vi "LINX - Servo Puerta 2.vi"() -> ()   [LabVIEW 2019]
doc: "This example demonstrates how to control a servo using LINX."
uses:
  <vilib>/MakerHub/LINX/Public/Utilities/Open Serial.vi
  <vilib>/MakerHub/LINX/Public/Sensors/Motion/Servo/Servo Open One Channel.vi
  <vilib>/MakerHub/LINX/Public/Sensors/Motion/Servo/Servo Set Pulse Width One Channel.vi
  <vilib>/MakerHub/LINX/Public/Sensors/Motion/Servo/Servo Close One Channel.vi
  <vilib>/MakerHub/LINX/LMH-LINX.lvlib
  <vilib>/MakerHub/LINX/Public/Sensors/Motion/Servo/Servo.lvlib
panel:
  out "Loop Rate (Hz)":u32
  in  "Cerrar":bool
  in  "Abrir":bool
  in  "Servo Channel":u8=2
  in  "Stop Button":bool
  in  "Serial Port":refnum<visa-resource-name>
  # "Servo Position \n(Pulse Width uS)"
  # "LINX Device Settings"
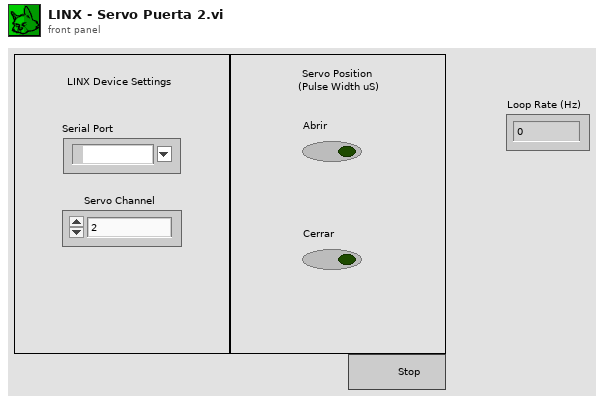
[diagram p1: front panel]
types:
  T1 = typedef "LMH-LINX.lvlib/LINX Ref.ctl" = cluster{"IO":T2, "Interface":T3, "LINX Device Config":T4}
  T2 = typedef "LMH-LINX.lvlib/Platform.ctl" = enum16{"Remote", "Local"}
  T3 = typedef "LMH-LINX.lvlib/Interface.ctl" = enum16{"Serial", "TCP"}
  T4 = typedef "LMH-LINX.lvlib/Device.lvlib/LINX Device Config.ctl" = cluster{"Interface":T3, "COM Port":refnum<visa-resource-name>, "TCP Configuration":T5, "Device Family":u8, "Device ID":u8, "Device Name":string, "TCP Ref":refnum<k5>, "Channels":T6}
  T5 = typedef "LMH-LINX.lvlib/Device.lvlib/TCP Config.ctl" = cluster{"IP Address":string, "Port":u16}
  T6 = typedef "LMH-LINX.lvlib/Channels.ctl" = cluster{"DI":u8[], "DO":u8[], "AI":u8[], "AO":u8[], "PWM":u8[], "QE":u8[], "UART":u8[], "I2C 2":u8[], "SPI":u8[], "CAN":u8[], "Servo":u8[], "AI Ref (V)":dbl, "AI Resolution (Bits)":u8, "AO Ref (V)":dbl, "AO Resolution (Bits)":u8}
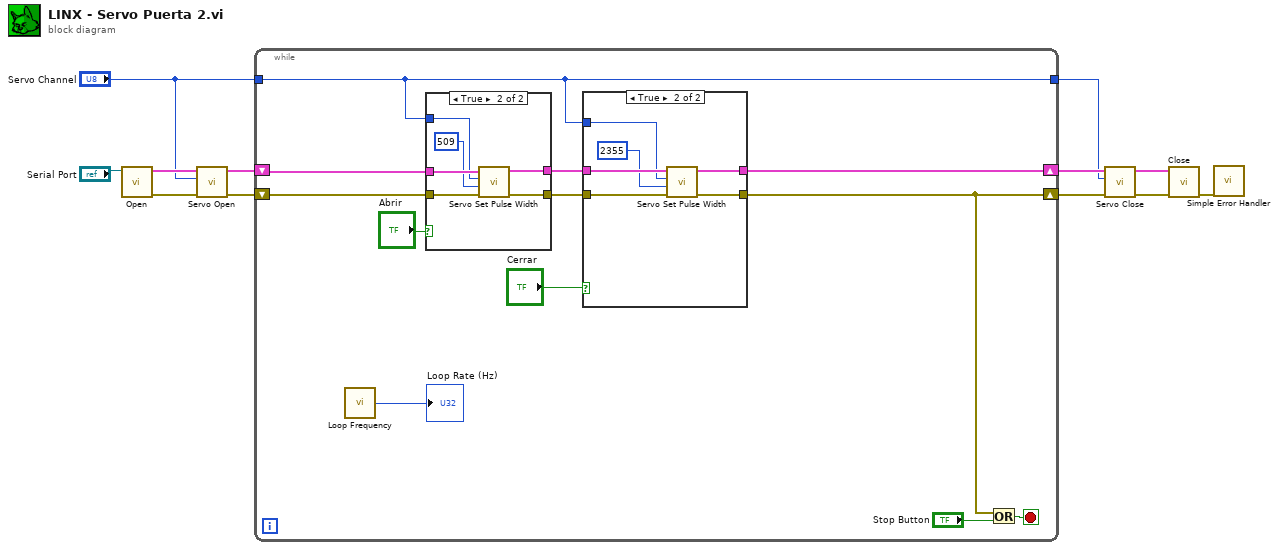
[diagram p0: block diagram]
diagram:
  n1 = call-poly <vilib>:"Open.vi"("Serial Port"="Serial Port") -> ("Error Out"=w11:errorcluster, "LINX Resource"=w10:T1)  [unwired: 8 in, 1 out]
  n2 = call-poly <vilib>:"Servo Open.vi"("Error In"=w11, "Servo Channel"="Servo Channel", "LINX Resource"=w10) -> ("Error Out"=w9:errorcluster, "LINX Resource"=w8:T1)  [unwired: 7 in]
  n3 = while {
    shift-right: [w15] -> w2
    shift-left: w9 -> [w22]
    tunnel: "Servo Channel" -> [w17]
    shift-right: [w19] -> w5
    shift-left: w8 -> [w21]
    tunnel: [w17] -> w1
    stop <- w24 stop-if-true
    n4 = call <vilib>:"Loop Frequency.vi"() -> ("Loop Rate (Hz)"=→"Loop Rate (Hz)":u32)
    n5 = case shown="True" "Abrir" {
      tunnel: w22 -> [w33 w40]
      tunnel: [w33 w39] -> w16
      tunnel: w21 -> [w34 w38]
      tunnel: [w34 w37] -> w18
      tunnel: w17 -> [_ w36]
      frame False {
      }
      frame True {
        n6 = call-poly <vilib>:"Servo Set Pulse Width.vi"("Error In"=w40, "Pulse Width (uS)"=509, "Servo Channel"=w36, "LINX Resource"=w38) -> ("Error Out"=w39:errorcluster, "LINX Resource"=w37:T1)  [unwired: 6 in]
      }
    }
    n7 = case shown="True" "Cerrar" {
      tunnel: w16 -> [w25 w32]
      tunnel: [w25 w31] -> w15
      tunnel: w18 -> [w26 w30]
      tunnel: [w26 w29] -> w19
      tunnel: w17 -> [_ w28]
      frame False {
      }
      frame True {
        n8 = call-poly <vilib>:"Servo Set Pulse Width.vi"("Error In"=w32, "Pulse Width (uS)"=2355, "Servo Channel"=w28, "LINX Resource"=w30) -> ("Error Out"=w31:errorcluster, "LINX Resource"=w29:T1)  [unwired: 6 in]
      }
    }
    n9 = Or(x=w15, y="Stop Button") -> (x .or. y?=w24:bool)
  }
  n10 = call-poly <vilib>:"Servo Close.vi"("Error In"=w2, "Servo Channel"=w1, "LINX Resource"=w5) -> ("Error Out"=w3:errorcluster, "LINX Resource"=w4:T1)  [unwired: 7 in]
  n11 = call <vilib>:"Close.vi"("Error In"=w3, "LINX Resource"=w4) -> ("Error Out"=w6:errorcluster)  [unwired: 9 in]
  n12 = call <vilib>:"Simple Error Handler.vi"("error in (no error)"=w6) -> ()  [unwired: 4 in, 5 out]
